vi "WPI_SerialPortQueryHubPaths.vi"(8 "error in (no error)":errorcluster) -> (0 "error out":errorcluster, 1 "Hub Path":string[](array[string]), 2 "OS Resource":string[](array[string]), 3 "VISA Resource":string[](array[string]))   [LabVIEW 2017]
uses:
  <vilib>/regexp/Match Regular Expression.xnode
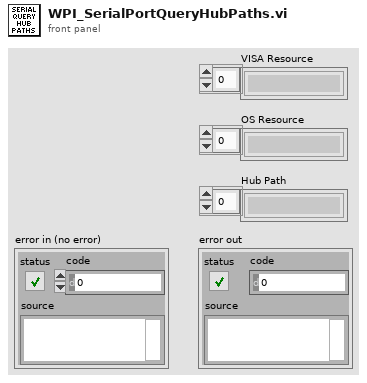
[diagram p1: front panel]
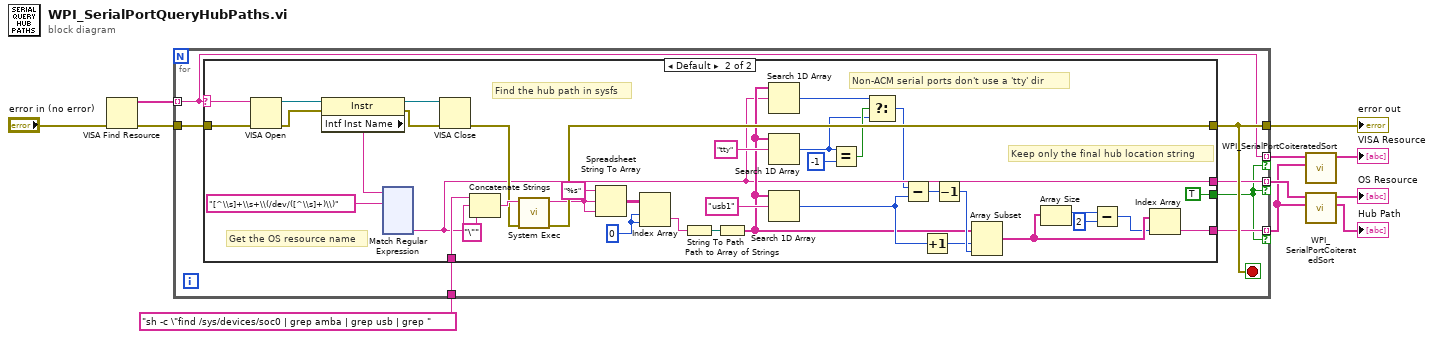
[diagram p0: block diagram]
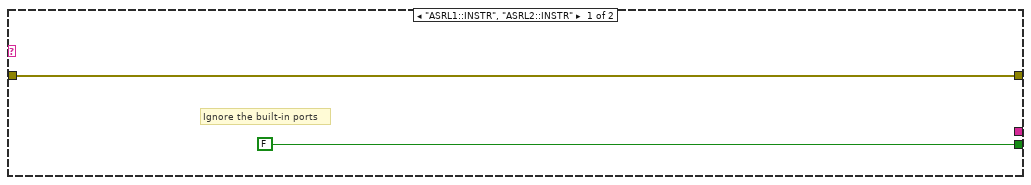
[diagram p2: hidden frame]
diagram:
  n1 = VISA Find Resource(8:"error in (no error)") -> (0:w10:errorcluster, 3:w7:string[])  [unwired: 2 in, 1 out]
  n2 = for {
    tunnel: w7 -> [w15] mode=indexing
    tunnel: [w18] -> w9
    tunnel: w10 -> [w17]
    tunnel: [w16] -> w6 mode=indexing if=w12
    tunnel: [w15] -> w2 mode=indexing if=w12
    tunnel: "sh -c \"find /sys/devices/soc0 | grep amba | grep usb | grep " ("command line") -> [w14]
    tunnel: [w13] -> w3 mode=indexing if=w12
    stop <- w18 stop-if-true
    n3 = case shown="Default" w15 {
      selector: w15 -> [_ w53]
      tunnel: [w20 w46] -> w18
      tunnel: w17 -> [w20 w56]
      tunnel: [_ w26] -> w16
      tunnel: [FALSE TRUE] -> w12
      tunnel: w14 -> [_ w48]
      tunnel: [_ w30] -> w13
      frame "ASRL1::INSTR", "ASRL2::INSTR" {
        # "Ignore the built-in ports"
      }
      frame Default {
        w42 = 0 ("disabled index (col)")
        # "Non-ACM serial ports don't use a 'tty' dir"
        # "Keep only the final hub location string"
        # "Find the hub path in sysfs"
        # "Get the OS resource name"
        n4 = VISA Open(error in (no error)=w56, VISA resource name=w53) -> (VISA resource name=w58:refnum<visa-resource-name>, error out=w55:errorcluster)  [unwired: 1 in, 2 out]
        n5 = property class="Instr"(reference=w58, error in=w55) -> (reference out=w57:refnum<visa-resource-name>, error out=w54:errorcluster, "Intf Inst Name"=w51:string)
        n6 = xnode "Match Regular Expression"("input string"=w51, "regular expression"="[^\\s]+\\s+\\(/dev/([^\\s]+)\\)") -> ("submatch 1"=w26:string)  [unwired: 4 in, 5 out]
        n7 = VISA Close(VISA resource name=w57, error in (no error)=w54) -> (error out=w47:errorcluster)
        n8 = Concatenate Strings(w48, w26, "\"" ("string")) -> (w49:string)
        n9 = call <vilib>:"System Exec.vi"("error in (no error)"=w47, "command line"=w49) -> ("error out"=w46:errorcluster, "standard output"=w43:string)  [unwired: 6 in, 2 out]
        n10 = Spreadsheet String To Array(format string="%s", spreadsheet string=w43, array type (2D Dbl)=w43) -> (array=w44:string[][])  [unwired: 1 in]
        n11 = Index Array(array=w44, index (row)=w42, index (col)=w42) -> (element=w28:string)
        n12 = String To Path(string=w28) -> (path=w40:path)
        n13 = Path to Array of Strings(0:w40) -> (2:w27:string[])  [unwired: 1 out]
        n14 = Search 1D Array(1D array=w27, element=w26) -> (index of element=w23:i32)  [unwired: 1 in]
        n15 = Search 1D Array(1D array=w27, element="tty") -> (index of element=w22:i32)  [unwired: 1 in]
        n16 = Search 1D Array(1D array=w27, element="usb1") -> (index of element=w36:i32)  [unwired: 1 in]
        n17 = Equal?(x=w22, y=-1) -> (x = y?=w24:bool)
        n18 = Select(t=w23, s=w24, f=w22) -> (s? t:f=w21:i32)
        n19 = Subtract(x=w21, y=w36) -> (x-y=w37:i32)
        n20 = Increment(x=w36) -> (x+1=w34:i32)
        n21 = Decrement(x=w37) -> (x-1=w35:i32)
        n22 = Array Subset(array=w27, index=w34, length=w35) -> (w33:string[])
        n23 = Array Size(array=w33) -> (size(s)=w32:i32)
        n24 = Subtract(x=w32, y=2) -> (x-y=w29:i32)
        n25 = Index Array(array=w33, index=w29) -> (element=w30:string)
      }
    }
  }
  "error out" <- w9
  n26 = call <vilib>:"WPI_SerialPortCoiteratedSort.vi"("Array to Sort"=w3, "Coiterated Array"=w2) -> ("Coiterated Array Out"=→"VISA Resource":string[])  [unwired: 8 in, 1 out]
  n27 = call <vilib>:"WPI_SerialPortCoiteratedSort.vi"("Array to Sort"=w3, "Coiterated Array"=w6) -> ("Sorted Array"=→"Hub Path":string[], "Coiterated Array Out"=→"OS Resource":string[])  [unwired: 8 in]
